vi "Process_SpectralEmissionGateSweep.vi"(0 "Refnum in":refnum<k34>, 1 "Acquire":bool, 2 "Capture number":i32, 5 "Gate Start":dbl, 7 "Gate Width":dbl, 9 "Image":dbl[][][](array[numeric]), 11 "error in (no error)":errorcluster, 12 "seconds since 1Jan1904":timestamp) -> (4 "Refnum out":refnum<k34>, 6 "Gate Delay Array":dbl[](array[numeric]), 8 "Avg Power each frame":dbl[](array[numeric]), 10 "Gate Delay of peak intensity":dbl, 15 "error out":errorcluster)   [LabVIEW 2017]
uses:
  <vilib>/Analysis/baseanly.llb/Mean (DBL).vi
  <vilib>/Analysis/NI_AALBase.lvlib
panel:
  in  "length":i32
  in  "index":i32
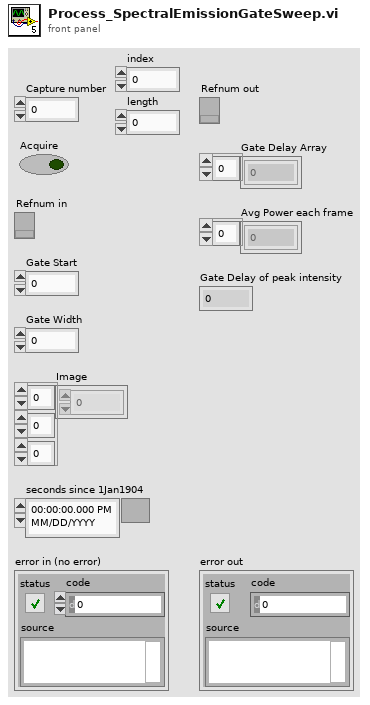
[diagram p1: front panel]
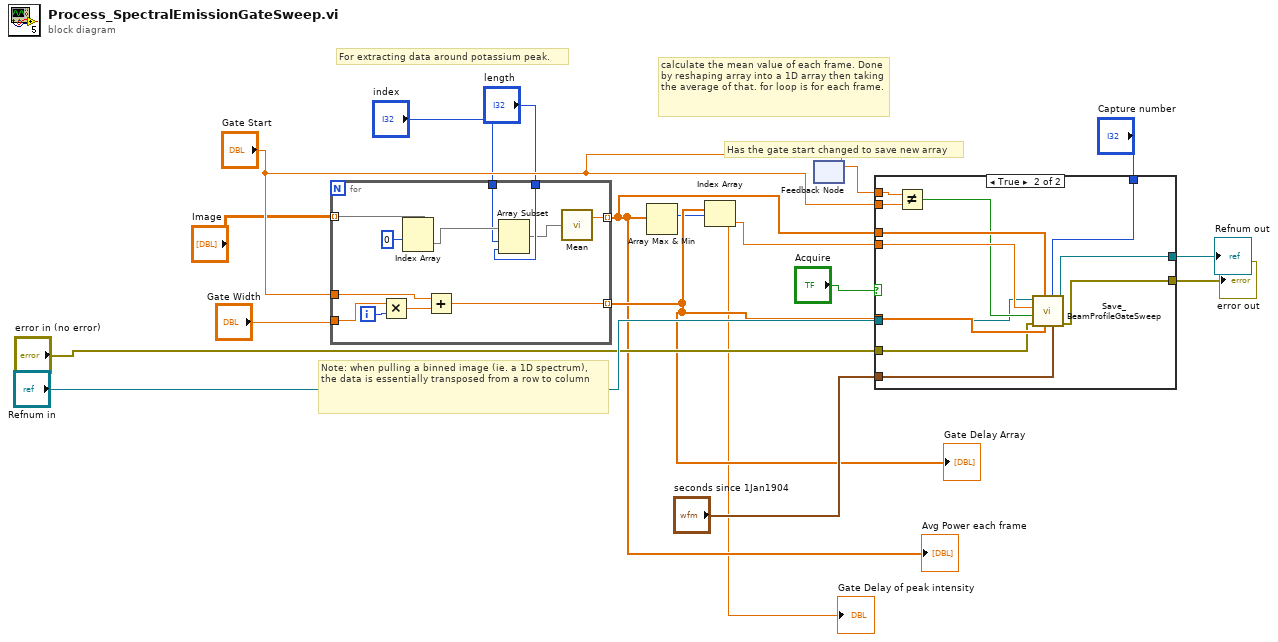
[diagram p0: block diagram]
diagram:
  # "For extracting data around potassium peak."
  # "Has the gate start changed to save new array"
  # "Note: when pulling a binned image (ie. a 1D spectrum), the data is essentially transposed from a row to column"
  # "calculate the mean value of each frame. Done by reshaping array into a 1D array then taking the average of that. for loop is for each frame."
  n1 = for {
    tunnel: "Image" -> [w23] mode=indexing
    tunnel: [w29] -> w7 mode=indexing
    tunnel: "Gate Start" -> [w25]
    tunnel: "Gate Width" -> [w27]
    tunnel: [w24] -> w8 mode=indexing
    tunnel: "index" -> [w20]
    tunnel: "length" -> [w19]
    i -> [w28]
    n2 = Multiply(x=w27, y=w28) -> (x*y=w26:dbl)
    n3 = Index Array(array=w23, index (row)=0) -> (element=w21:dbl[])  [unwired: 1 in]
    n4 = Add(x=w25, y=w26) -> (x+y=w24:dbl)
    n5 = Array Subset(array=w21, index=w20, length=w19) -> (w18:dbl[])
    n6 = call-poly <vilib>:"Mean.vi"("X"=w18) -> ("mean"=w29:dbl)  [unwired: 1 out]
  }
  "Gate Delay Array" <- w8
  "Avg Power each frame" <- w7
  n7 = Array Max & Min(array=w7) -> (max index (indices)=w4:i32)  [unwired: 3 out]
  n8 = Index Array(array=w8, index=w4) -> (element=w5:dbl)
  "Gate Delay of peak intensity" <- w5
  n9 = feedback #1() -> (w11:dbl)  [unwired: 1 in]
  n10 = feedback-in #1("Gate Start") -> ()
  n11 = case shown="True" "Acquire" {
    tunnel: "seconds since 1Jan1904" -> [_ w38]
    tunnel: "Capture number" -> [_ w43]
    tunnel: w5 -> [_ w42]
    tunnel: w7 -> [_ w41]
    tunnel: w8 -> [_ w40]
    tunnel: w11 -> [_ w37]
    tunnel: "Gate Start" -> [_ w36]
    tunnel: [w30 w35] -> w14
    tunnel: [w31 w34] -> w15
    tunnel: "error in (no error)" -> [w30 w33]
    tunnel: "Refnum in" -> [w31 w32]
    frame False {
    }
    frame True {
      n12 = Not Equal?(x=w37, y=w36) -> (x != y?=w39:bool)
      n13 = call "Save_BeamProfileGateSweep.vi"("TimeStamp"=w38, "Capture Number"=w43, "Gate Delay Array"=w40, "Average power"=w41, "Error In"=w33, "Save new Gate delay array"=w39, "Gate Delay of peak intensity"=w42, "File In"=w32) -> ("error out"=w35:errorcluster, "File Out"=w34:refnum<k34>)  [unwired: 2 in]
    }
  }
  "Refnum out" <- w15
  "error out" <- w14
